vi "Write GoogleAPI URI.vi"(8 "error in (no error)":errorcluster, 10 "Token Server URI":string, 11 "Oauth2.Google in":refnum<class "Oauth2.Google.lvclass">) -> (0 "error out":errorcluster, 3 "Oauth2.Google out":refnum<class "Oauth2.Google.lvclass">)   [LabVIEW 2013, in "Oauth2.Google.lvclass"]
uses:
  Oauth2.Google.lvclass
  Oauth2.Google.lvclass/Oauth2.Google.ctl
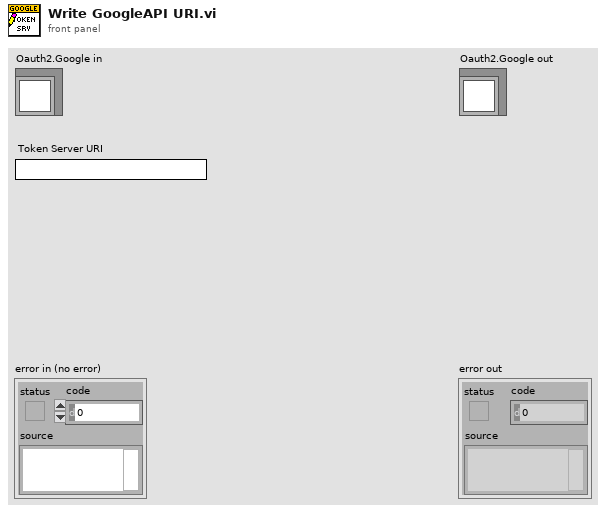
[diagram p1: front panel]
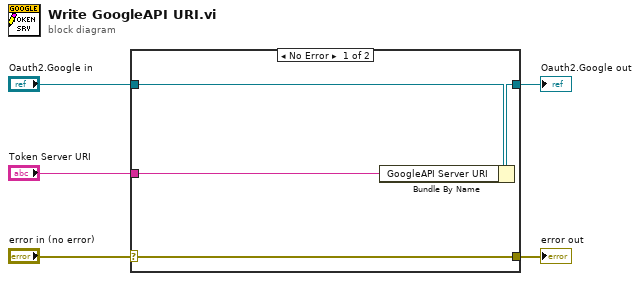
[diagram p0: block diagram]
diagram:
  n1 = case shown="No Error" "error in (no error)" {
    selector: "error in (no error)" -> [w9 w10]
    tunnel: [w9 w10] -> w4
    tunnel: [w7 w11] -> w2
    tunnel: "Oauth2.Google in" -> [w8 w11]
    tunnel: "Token Server URI" -> [w6 _]
    frame No Error {
      n2 = Bundle By Name(cluster=w8, "GoogleAPI Server URI"=w6) -> (w7:refnum<class "Oauth2.Google.lvclass">)
    }
    frame Error {
    }
  }
  "error out" <- w4
  "Oauth2.Google out" <- w2
